vi "globalVariables.vi"() -> ()   [LabVIEW 2012]
uses:
  TimeValue.ctl
  SensorSettingCtl.ctl
panel:
  in  "Path for measuring results":path=path "C:/Users/Induelec/Desktop/test_output"
  out "Program running":bool[](array[boolean])
  out "AllValuesSemaphore":T1
  in  "stop measurement":bool
  out "Saved Configuration":T2[](array[typedef])
  in  "AllValues":T3[][](array[typedef])
  in  "NewestValues":T3[](array[typedef])=[{"Time of measurement"=timestamp(0 s since 1904-01-01), "Current value"=0.0}, {"Time of measurement"=timestamp(0 s since 1904-01-01), "Current value"=0.0}, {"Time of measurement"=timestamp(0 s since 1904-01-01), "Current value"=0.0}, {"Time of measurement"=timestamp(0 s since 1904-01-01), "Current value"=0.0}, {"Time of measurement"=timestamp(0 s since 1904-01-01), "Current value"=0.0}]
  in  "MaxNrOfChannels":i32=5
  out "Errors":errorcluster[](array[cluster])
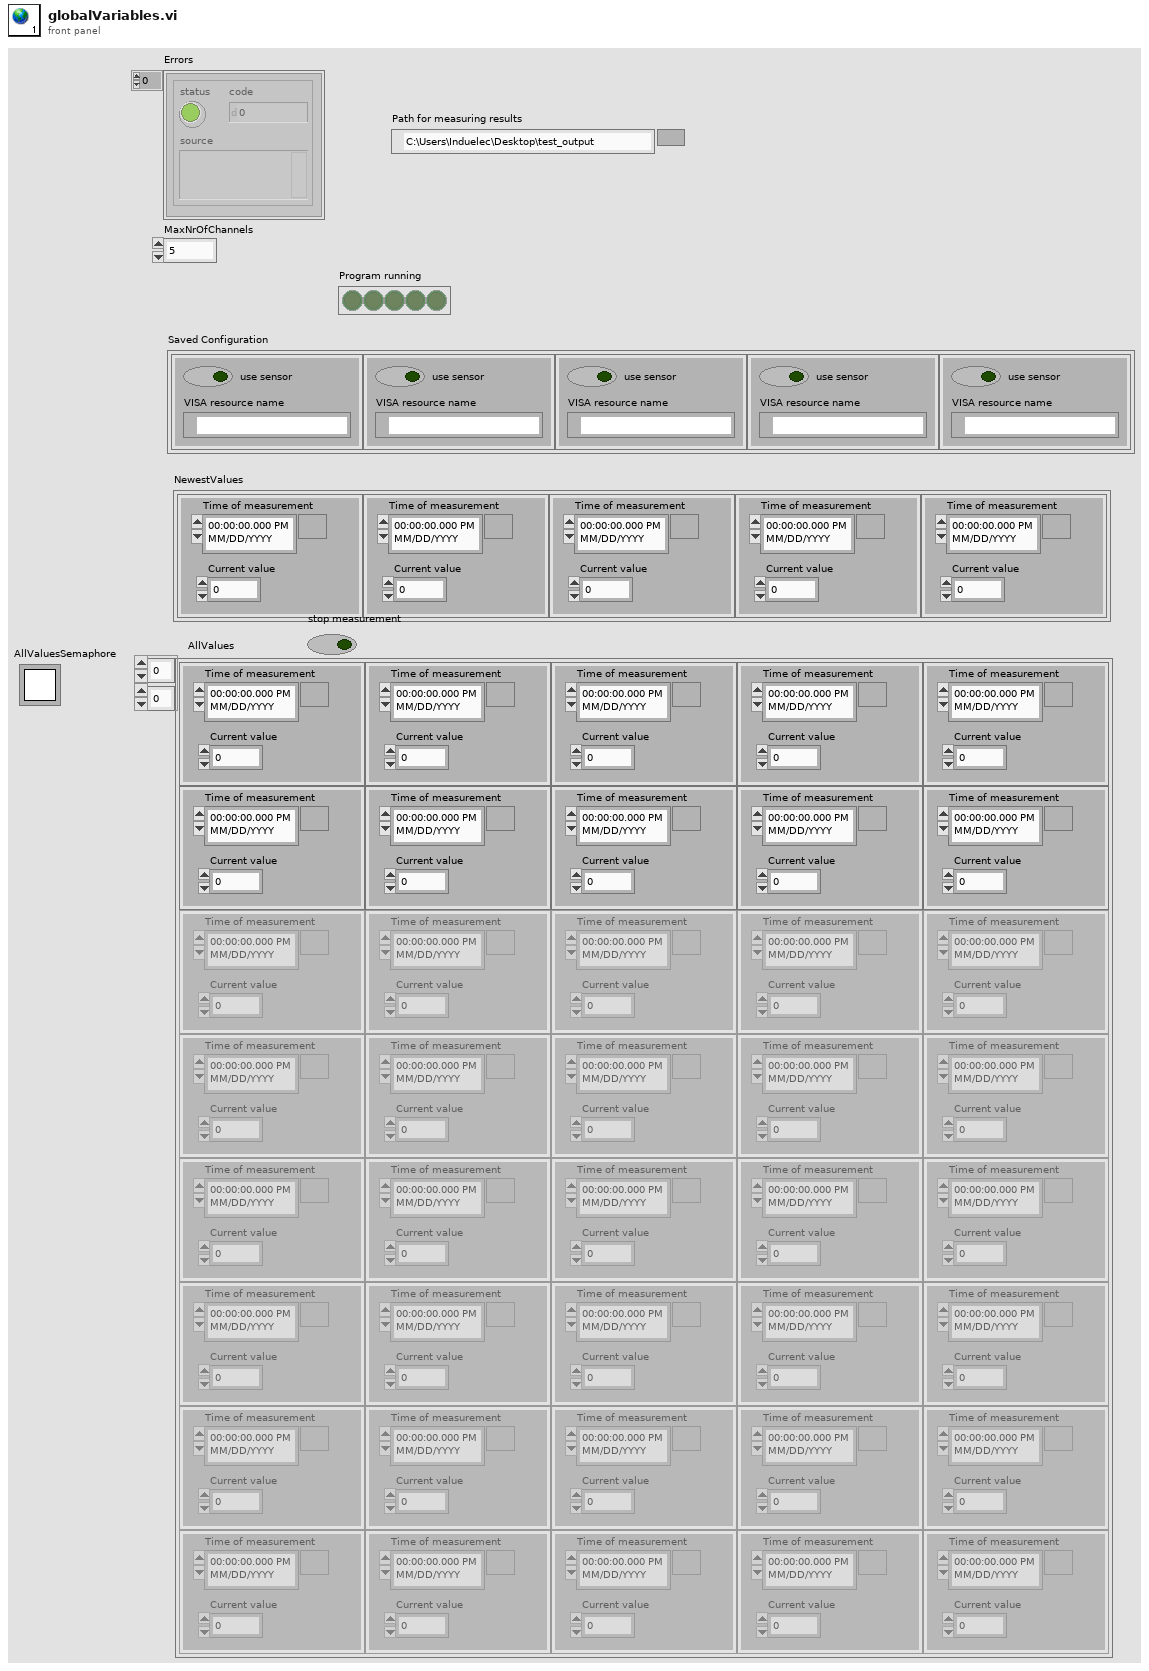
[diagram p1: front panel]
types:
  T1 = typedef "Semaphore RefNum" = refnum<k1>
  T2 = typedef "SensorSettingCtl.ctl" = cluster{"VISA resource name":refnum<visa-resource-name>, "use sensor":bool}
  T3 = typedef "TimeValue.ctl" = cluster{"Time of measurement":timestamp, "Current value":dbl}
diagram:
